vi "Read Limit Test Type.vi"(8 "error in (no error)":errorcluster, 11 "Test Double Float in":refnum<class "Test Double Float.lvclass">) -> (0 "error out":errorcluster, 2 "Limit Test Type":T1, 3 "Test Double Float out":refnum<class "Test Double Float.lvclass">)   [LabVIEW 2021, in "BT.lvlib" / "Test Double Float.lvclass"]
uses:
  Test Double Float.lvclass
  Support/Limit Test Type.ctl
  Test Double Float.lvclass/Test Double Float.ctl
  BT.lvlib
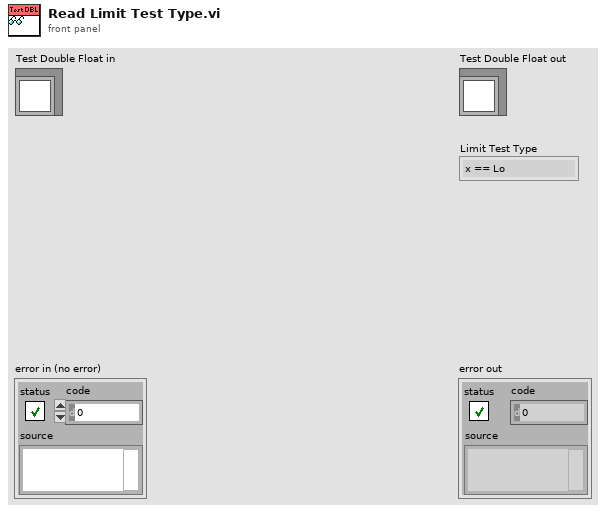
[diagram p1: front panel]
types:
  T1 = typedef "BT.lvlib/Limit Test Type.ctl" = enum16{"x == Lo", "x != Lo", "x > Lo", "x < Lo", "x >= Lo", "x <= Lo", "Lo > x < Hi", "Lo >= x <= Hi", "Lo >= x < Hi", "Lo > x <= Hi", "Lo < x > Hi", "Lo <= x >= Hi", "Lo <= x > Hi", "Lo < x >= Hi", "x == Lo +/- Hi"}
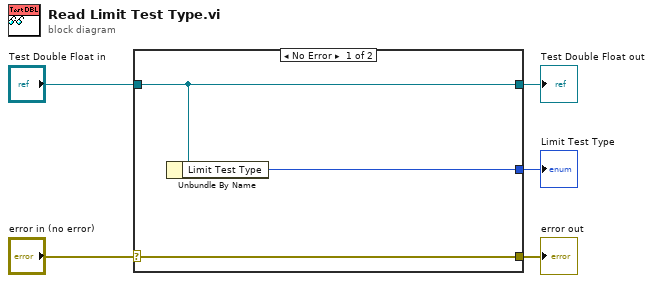
[diagram p0: block diagram]
diagram:
  n1 = case shown="No Error" "error in (no error)" {
    selector: "error in (no error)" -> [w8 w9]
    tunnel: [w8 w9] -> w4
    tunnel: [w7 w10] -> w2
    tunnel: "Test Double Float in" -> [w7 w10]
    tunnel: [w6 _] -> w1
    frame No Error {
      n2 = Unbundle By Name(w7) -> ("Limit Test Type"=w6:T1)
    }
    frame Error {
    }
  }
  "error out" <- w4
  "Test Double Float out" <- w2
  "Limit Test Type" <- w1
